vi "Actor Core.vi"(8 "error in":errorcluster, 11 "Data Viewer in":refnum<class "Task Viewer.lvclass">) -> (0 "error out":errorcluster, 3 "Actor out":refnum<class "Actor.lvclass">)   [LabVIEW 2020, in "Task Viewer.lvlib" / "Task Viewer.lvclass"]
doc: "The user interface for this panel.\n----\nCopyright: MGI 2016\nAuthor: Derek Trepanier"
uses:
  Task Viewer.lvclass
  C:/Program Files/National Instruments/LabVIEW 2020/vi.lib/MGI/Panel Manager/Panel Actor/Panel Actor/Panel Actor.lvclass
  <vilib>/ActorFramework/Actor/Actor.lvclass
  Task Viewer.lvclass/Task Viewer.ctl
  Task Viewer enum df.ctl
  <vilib>/MGI/Panel Manager/Panel Actor/Panel Actor/Panel Actor.lvclass
panel:
  out "Countdown":string
  out "Waveform Chart":T1(graph)
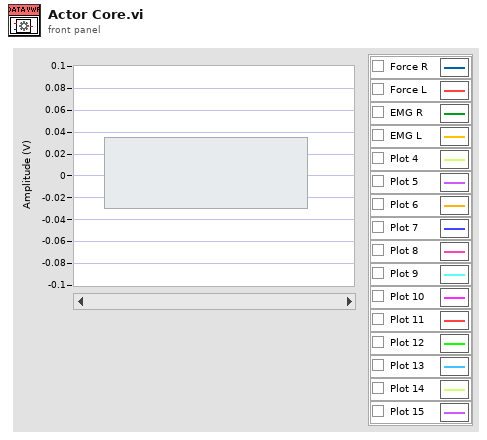
[diagram p1: front panel]
types:
  T1 = cluster{"Disp Data[0]":dbl, "Disp Data[1]":dbl, "Disp Data[2]":dbl, "Disp Data[3]":dbl, "Disp Data[4]":dbl, "Disp Data[5]":dbl, "Disp Data[6]":dbl, "Disp Data[7]":dbl, "Disp Data[8]":dbl, "Disp Data[9]":dbl, "Disp Data[10]":dbl, "Disp Data[11]":dbl, "Disp Data[12]":dbl, "Disp Data[13]":dbl, "Disp Data[14]":dbl, "Disp Data[15]":dbl}
  T2 = cluster{"Event Registration Refnum":refnum<event-registration>, "Pnl Actor":refnum<event-registration>}
  T3 = cluster{"Disp Data[0]":dbl, "Disp Data[1]":dbl, "Disp Data[2]":dbl, "Disp Data[3]":dbl, "Disp Data[4]":dbl, "Disp Data[5]":dbl, "Disp Data[6]":dbl, "Disp Data[7]":dbl, "Disp Data[8]":dbl, "Disp Data[9]":dbl, "Disp Data[10]":dbl, "Disp Data[11]":dbl, "Disp Data[12]":dbl, "Disp Data[13]":dbl, "Disp Data[14]":dbl, "Disp Data[15]":dbl}[]
  T4 = typedef "Task Viewer enum df.ctl" = enum16{"Idle", "Countdown", "Close Helper"}
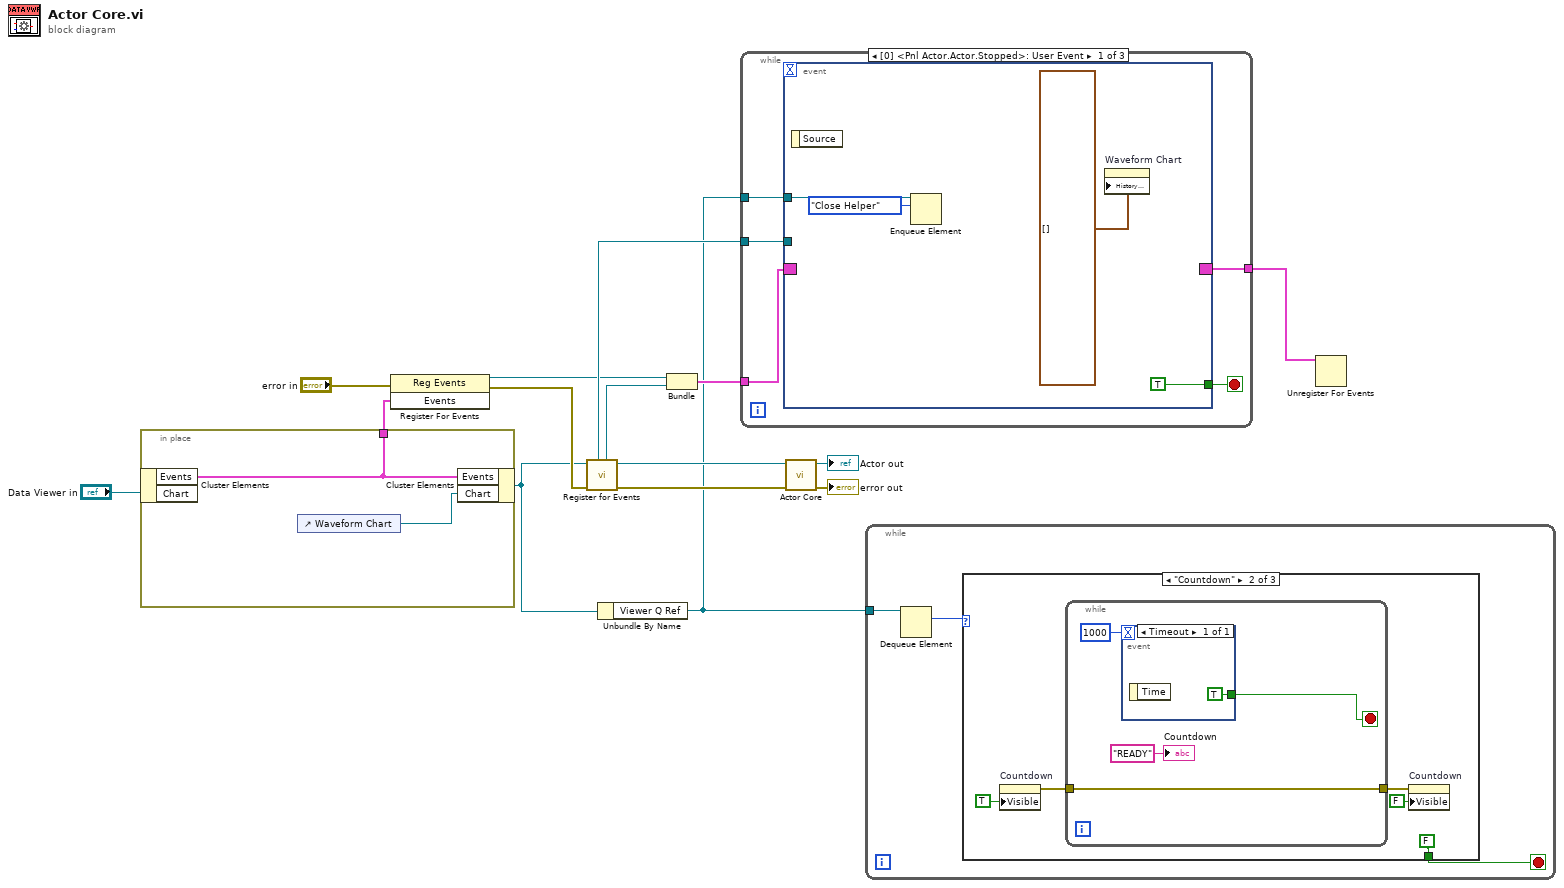
[diagram p0: block diagram]
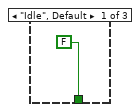
[diagram p2: hidden frame]
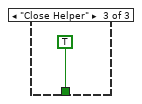
[diagram p3: hidden frame]
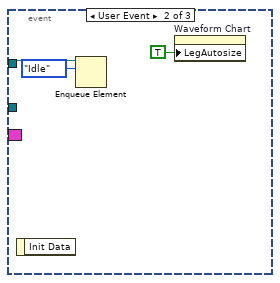
[diagram p4: hidden frame]
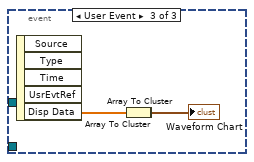
[diagram p5: hidden frame]
diagram:
  n1 = in-place {
    in-place-border: [w17] -> w9
    n2 = in-place-cluster #1("Data Viewer in") -> ("Events"=w17:cluster{"Update Plot":refnum<user-event>})  [unwired: 1 out]
    n3 = control-ref of="Waveform Chart"() -> (w16:refnum<vi>)
    n4 = in-place-cluster #1("Events"=w17, "Chart"=w16) -> (w2:refnum<class "Task Viewer.lvclass">)
  }
  n5 = register-events(error in="error in", w9) -> (reference out=w6:refnum<event-registration>, error out=w7:errorcluster)  [unwired: 1 in]
  n6 = call <vilib>:"Register for Events.vi"("Error In"=w7, "Panel Actor in"=w2) -> ("Error Out"=w13:errorcluster, "Panel Actor out"=w12:refnum<class "Task Viewer.lvclass">, "Pnl Actor"=w5:refnum<event-registration>, "Self Enqueuer"=w11:refnum<class "Message Enqueuer.lvclass">)  [unwired: 6 in]
  n7 = Unbundle By Name(w2) -> ("Viewer Q Ref"=w1:refnum<queue>)
  n8 = Bundle("Event Registration Refnum"=w6, "Pnl Actor"=w5) -> (w4:T2)  [unwired: 1 in]
  n9 = while {
    tunnel: w11 -> [w21]
    tunnel: w4 -> [w20]
    tunnel: [w19] -> w3
    tunnel: w1 -> [w18]
    stop <- w22 stop-if-true
    n10 = event shown="[0] <Pnl Actor.Actor.Stopped>: User Event" {
      selector: w20 -> [_ _ _]
      dyn-events: [_ _ _] -> w19
      timeout: _ -> [_ _ _]
      tunnel: [TRUE _ _] -> w22
      tunnel: w21 -> [_ _ _]
      tunnel: w18 -> [w25 w28 _]
      event User Event {
        n11 = event-data() -> ()  [unwired: 1 in, 1 out]
        n12 = Enqueue Element(queue=w25, element=Task_Viewer_enum_df."Close Helper") -> ()  [unwired: 2 in, 3 out]
        n13 = property on="Waveform Chart" class="WFChart (strict)"("History Data"=T3 []) -> ()  [unwired: 2 in, 2 out]
      }
      event User Event {
        n14 = event-data() -> ()  [unwired: 1 in, 1 out]
        n15 = Enqueue Element(queue=w28, element=Task_Viewer_enum_df."Idle") -> ()  [unwired: 2 in, 3 out]
        n16 = property on="Waveform Chart" class="WFChart (strict)"("LegAutosize"=TRUE ("Legend:Autosize")) -> ()  [unwired: 2 in, 2 out]
      }
      event User Event {
        n17 = event-data() -> ("Disp Data"=w30:dbl[])  [unwired: 1 in, 4 out]
        n18 = Array To Cluster(array=w30) -> ()  [unwired: 1 out]
        n19 = Array To Cluster(array=w30) -> (cluster=→"Waveform Chart":T1)
      }
    }
  }
  n20 = call-parent "Actor Core.vi"("error in"=w13, "Panel Actor in"=w12) -> ("error out"=→"error out":errorcluster, "Actor out"=→"Actor out":refnum<class "Actor.lvclass">)  [unwired: 8 in]
  n21 = while {
    tunnel: w1 -> [w34]
    stop <- w32 stop-if-true
    n22 = Dequeue Element(queue=w34) -> (element=w33:T4)  [unwired: 2 in, 3 out]
    n23 = case shown="\"Countdown\"" w33 {
      tunnel: [FALSE FALSE TRUE] -> w32
      frame "Idle", Default {
      }
      frame "Countdown" {
        n24 = property on="Countdown" class="Str"("Visible"=TRUE) -> (error out=w38:errorcluster)  [unwired: 2 in, 1 out]
        n25 = while {
          tunnel: w38 -> [w42]
          tunnel: [w42] -> w36
          stop <- w41 stop-if-true
          n26 = event shown="[0] Timeout" {
            selector: _ -> [_]
            dyn-events: _ -> [_]
            timeout: 1000 -> [_]
            tunnel: [TRUE] -> w41
            event Timeout {
              n27 = event-data() -> ()  [unwired: 1 in, 1 out]
            }
          }
          "Countdown" <- "READY" ("Countdown")
        }
        n28 = property on="Countdown" class="Str"(error in=w36, "Visible"=FALSE) -> ()  [unwired: 1 in, 2 out]
      }
      frame "Close Helper" {
      }
    }
  }
  n29 = Unregister For Events(event registration refnum=w3) -> ()  [unwired: 1 in, 1 out]
